vi "BlockUpload.vi"() -> ()   [LabVIEW 2019]
uses:
  lib/Snap7.lvlib
panel:
  out "?":string
  in  "BlockType":i32(ring)=66 items=["OB"=56, "DB"=65, "SDB"=66, "FC"=67, "SFC"=68, "FB"=69, "SFB"=70]
  out "Hex Data":string
  out "Size Get":i32
  out "Running":bool
  out "Status":string="No Error"
  in  "Number":i32=1
  in  "?":bool
  in  "Slot":i32=2
  in  "Rack":i32
  in  "Address IP":string="192.168.1.12"
  # "Block"
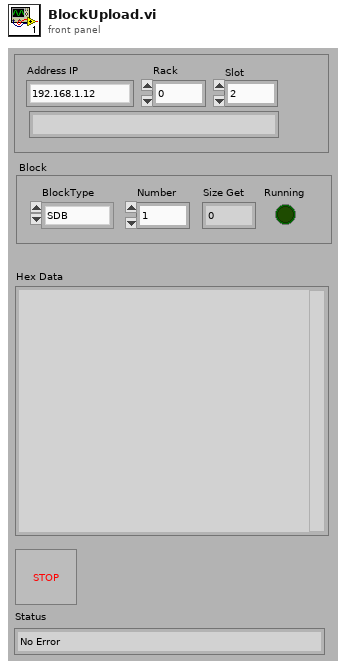
[diagram p1: front panel]
types:
  T1 = enum16{"big-endian, network order", "native, host order", "little-endian"}
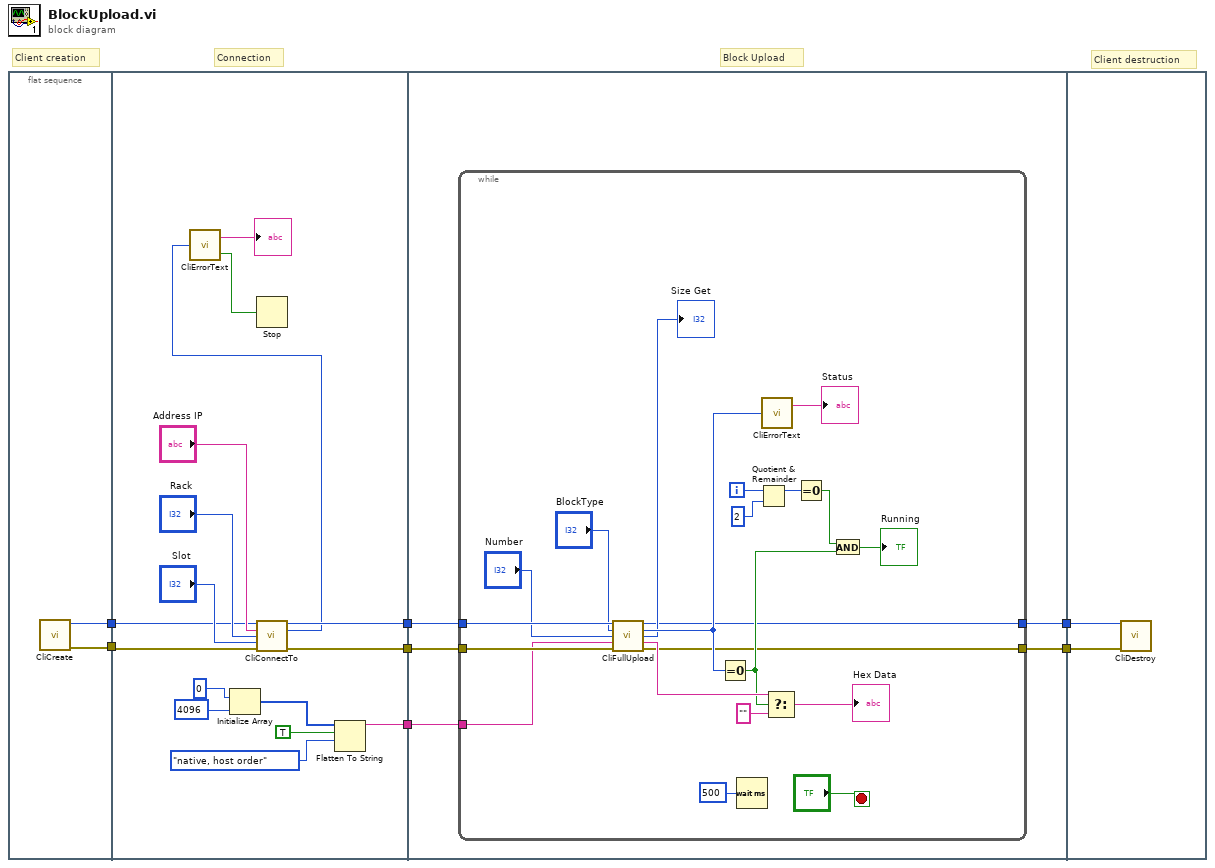
[diagram p0: block diagram]
diagram:
  # "Client destruction"
  # "Block Upload"
  # "Connection"
  # "Client creation"
  n1 = flat-sequence {
    tunnel: [w9] -> w4
    tunnel: [w8] -> w3
    tunnel: [w20] -> w7
    tunnel: [w13] -> w6
    tunnel: [w19] -> w5
    tunnel: w4 -> [w15]
    tunnel: w3 -> [w14]
    tunnel: w7 -> [w30]
    tunnel: w6 -> [w29]
    tunnel: w5 -> [w28]
    tunnel: [w27] -> w2
    tunnel: [w26] -> w1
    tunnel: w2 -> [w53]
    tunnel: w1 -> [w52]
    frame #0 {
      n2 = call "CliCreate.vi"() -> ("ref out"=w9:u64, "error out"=w8:errorcluster)  [unwired: 14 in]
    }
    frame #1 {
      n3 = Initialize Array(u8 0, 4096) -> (w23:u8[])
      n4 = call "CliConnectTo.vi"("ref in"=w15, "Address"="Address IP", "Rack"="Rack", "Slot"="Slot", "error in (no error)"=w14) -> ("ref out"=w13:u64, "Result"=w10:i32, "error out"=w20:errorcluster)  [unwired: 8 in]
      n5 = call "CliErrorText.vi"("ErrNo"=w10) -> ("Error"=w11:bool, "ErrMessage"=→"?":string)
      n6 = Stop(stop? (T)=w11) -> ()
      n7 = Flatten To String(anything=w23, prepend array or string size? (T)=TRUE, byte order (0:big-endian, network order)=T1."native, host order") -> (data string=w19:string)  [unwired: 1 in, 2 out]
    }
    frame #2 {
      n8 = while {
        tunnel: w30 -> [w42]
        tunnel: w29 -> [w44]
        tunnel: w28 -> [w39]
        tunnel: [w32] -> w27
        tunnel: [w31] -> w26
        i -> [w49]
        stop <- "?" stop-if-true
        n9 = call "CliFullUpload.vi"("ref in"=w44, "BlockType"="BlockType", "Block Number"="Number", "data in"=w39, "error in (no error)"=w42) -> ("ref out"=w32:u64, "Result"=w43:i32, "SizeGet"=→"Size Get":i32, "data out"=w41:string, "error out"=w31:errorcluster)  [unwired: 6 in]
        n10 = Equal To 0?(x=w43) -> (x = 0?=w33:bool)
        n11 = Wait (ms)(milliseconds to wait=u32 500 ("Loop Delay (ms)")) -> ()  [unwired: 1 out]
        n12 = Quotient & Remainder(x=w49, y=2) -> (x-y*floor(x/y)=w47:i32)  [unwired: 1 out]
        n13 = call "CliErrorText.vi"("ErrNo"=w43) -> ("ErrMessage"=→"Status":string)  [unwired: 1 out]
        n14 = Select(t=w41, s=w33, f="") -> (s? t:f=→"Hex Data":string)
        n15 = Equal To 0?(x=w47) -> (x = 0?=w46:bool)
        n16 = And(x=w46, y=w33) -> (x .and. y?=→"Running":bool)
      }
    }
    frame #3 {
      n17 = call "CliDestroy.vi"("ref in"=w53, "error in (no error)"=w52) -> ()  [unwired: 13 in, 1 out]
    }
  }
